vi "E15_TareaRaíces.vi"() -> ()   [LabVIEW 2026]
panel:
  out "Gráfica":cluster{dbl[], dbl[]}(graph)
  out "Tipo de raíz":string
  out "Raíz 2":string
  out "Raíz 1":string
  in  "Calcular":bool
  in  "c":dbl
  in  "b":dbl
  in  "a":dbl
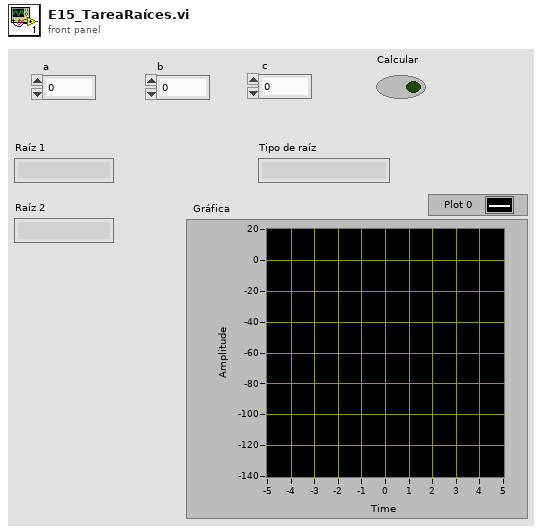
[diagram p1: front panel]
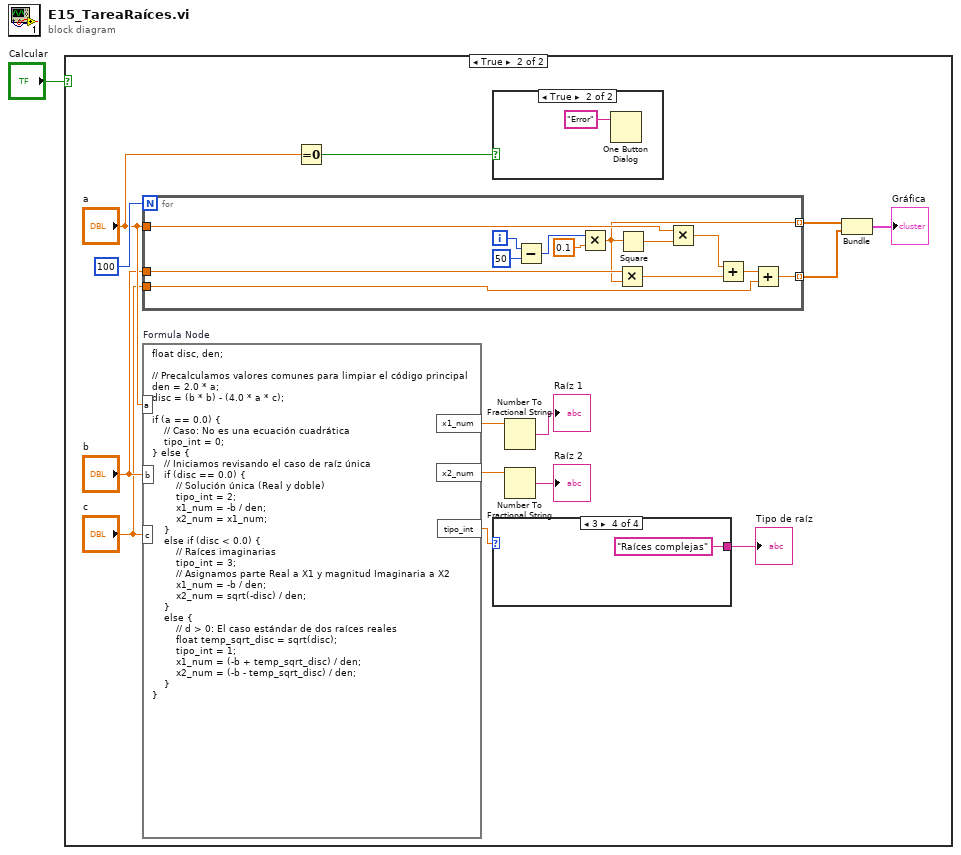
[diagram p0: block diagram]
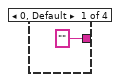
[diagram p4: hidden frame]
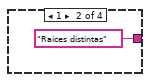
[diagram p5: hidden frame]
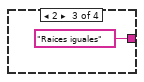
[diagram p6: hidden frame]
diagram:
  n1 = case shown="True" "Calcular" {
    frame False {
    }
    frame True {
      n2 = for {
        N: 100 -> [_]
        tunnel: [w21] -> w7 mode=indexing
        tunnel: [w16] -> w5 mode=indexing
        tunnel: "a" -> [w24]
        tunnel: "b" -> [w23]
        tunnel: "c" -> [w19]
        i -> [w28]
        n3 = Subtract(x=w28, y=50 ("x")) -> (x-y=w25:i32)
        n4 = Multiply(x=w25, y=0.1) -> (x*y=w21:dbl)
        n5 = Multiply(x=w23, y=w21) -> (x*y=w18:dbl)
        n6 = Square(x=w21) -> (x^2=w22:dbl)
        n7 = Multiply(x=w24, y=w22) -> (x*y=w20:dbl)
        n8 = Add(x=w20, y=w18) -> (x+y=w17:dbl)
        n9 = Add(x=w17, y=w19) -> (x+y=w16:dbl)
      }
      n10 = formula code="float disc, den;\n\n// Precalculamos valores comunes para limpiar el código principal\nden = 2.0 * a;\ndisc = (b * b) - (4.0 * a * c);\n\nif (a == 0.0) {\n    // Caso: No es una ecuación cuadrática\n    tipo_int = 0;\n} else {\n    // Iniciamos revisando el caso de raíz única\n    if (disc == 0.0) {\n        // Solución única (Real y doble)\n        tipo_int = 2;\n        x1_num = -b / den;\n        x2_num = x1_num;\n    }\n    else if (disc < 0.0) {\n        // Raíces imaginarias\n        tipo_int = 3;\n        // Asignamos parte Real a X1 y magnitud Imaginaria a X2\n        x1_num = -b / den;\n        x2_num = sqrt(-disc) / den;\n    }\n    else {\n        // d > 0: El caso estándar de dos raíces reales\n        float temp_sqrt_disc = sqrt(disc);\n        tipo_int = 1;\n        x1_num = (-b + temp_sqrt_disc) / den;\n        x2_num = (-b - temp_sqrt_disc) / den;\n    }\n}"("a"="a", "b"="b", "c"="c") -> ("x1_num"=w13:dbl, "x2_num"=w12:dbl, "tipo_int"=w11:dbl)
      n11 = Equal To 0?(x="a") -> (x = 0?=w10:bool)
      n12 = case shown="True" w10 {
        frame False {
        }
        frame True {
          n13 = One Button Dialog(message="Error") -> ()  [unwired: 1 in, 1 out]
        }
      }
      n14 = case shown="3" w11 {
        tunnel: ["" "Raíces distintas" "Raíces iguales" "Raíces complejas"] -> w9
        frame 0, Default {
        }
        frame 1 {
        }
        frame 2 {
        }
        frame 3 {
        }
      }
      "Tipo de raíz" <- w9
      n15 = Number To Fractional String(number=w13) -> (F-format string=→"Raíz 1":string)  [unwired: 3 in]
      n16 = Number To Fractional String(number=w12) -> (F-format string=→"Raíz 2":string)  [unwired: 3 in]
      n17 = Bundle "Bundle"(w7, w5) -> (→"Gráfica":cluster{dbl[], dbl[]})  [unwired: 1 in]
    }
  }
